vi "Check_Beam_Powers.vi"(3 "Mode":T7, 5 "Traverse line In":T4 {"Carrier_2 Q (l/min)" format="%#.2f"; "Row Duration (mins)" format="%#.1f"; "Row No" min=0; "Trace Gas Concentration (%)" min=0.0 format="%#_4f"; "Carrier_1 Q (l/min)" format="%#.2f"; "Tunnel Speed" format="%#.2f"; "Start X" format="%#.2f"; "Start Y" format="%#.2f"; "Start Z" format="%#.2f"; "End X" format="%#.2f"; "End Y" format="%#.2f"; "End Z" format="%#.2f"; "Averaging time (min)" min=0.0 format="%#.2f"}) -> (0 "Error Message":string, 1 "Status":T3, 2 "Traverse line Out":T4 {"Carrier_2 Q (l/min)" format="%#.2f"; "Row Duration (mins)" format="%#.1f"; "Row No" min=0; "Trace Gas Concentration (%)" min=0.0 format="%#_4f"; "Carrier_1 Q (l/min)" format="%#.2f"; "Tunnel Speed" format="%#.2f"; "Start X" format="%#.2f"; "Start Y" format="%#.2f"; "Start Z" format="%#.2f"; "End X" format="%#.2f"; "End Y" format="%#.2f"; "End Z" format="%#.2f"; "Averaging time (min)" min=0.0 format="%#.2f"})   [LabVIEW 2016]
uses:
  Gen Trav/Traverse_cluster.ctl
  Gen Trav/Spacing.ctl
  Controls/Multi_run_mode.ctl
  Controls/User_Specific_mode.ctl
  Gen Trav/Multi_Run_Status.ctl
  Controls/Beam_Type.ctl
  Gen Trav/Route mapping/Axis.ctl
  Globals/Meas_global.vi
  Globals/Extra_Commands_Global.vi
  Globals/LDA_meas_global_1.vi
panel:
  out "Power Chart":T1(graph)
  out "Light Power":dbl=8.10606551e-08 format="%^#_9e"
  in  "stop":bool
  out "Powers":dbl[](array[numeric]) format="%.1f"
  out "Beam Data":dbl[][](array[numeric]) format="%.1f"
  out "Beam Type":T2 items=["Green Unshifted", "Green Shifted", "Blue Unshifted", "Blue Shifted"]
  # "X                      Y                   Z"
  # "Green Unshifted\nGreen Shifted\nBlue Unshifted\nBlue Shifted"
  # "X           Y            Z"
  # "Start"
  # "End"
  # "X           Y            Z"
  # "Start"
  # "End"
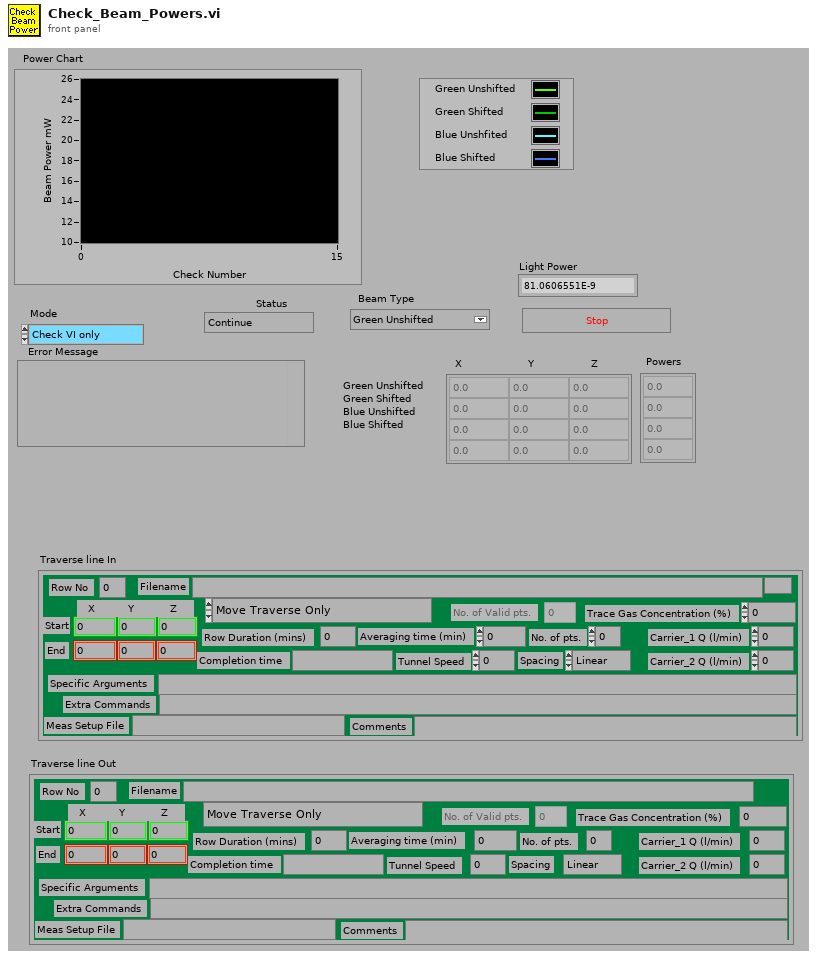
[diagram p1: front panel]
types:
  T1 = cluster{"Numeric":dbl, "Numeric":dbl, "Numeric":dbl, "Numeric":dbl}
  T2 = typedef "Beam_Type.ctl" = u16
  T3 = typedef "Multi_Run_Status.ctl" = enum16{"Continue", "Continue with Error", "Jump to Next Point", "Jump to Next Row", "Jump To Fall Back", "Terminate Run"}
  T4 = typedef "Traverse_cluster.ctl" = cluster{"Start X":sgl, "Start Y":sgl, "Start Z":sgl, "End X":sgl, "End Y":sgl, "End Z":sgl, "No. of pts.":i32, "Spacing":T5, "Filename":path, "Tunnel Speed":dbl, "Averaging time (min)":dbl, "Extra Commands":string, "Carrier_1 Q (l/min)":dbl, "Carrier_2 Q (l/min)":dbl, "Trace Gas Concentration (%)":dbl, "Specific Arguments":string, "Comments":string, "Row No":i32, "Row Type Selector":T6, "Completion time":string, "Row Duration (mins)":dbl, "No. of Valid pts.":i32, "Meas Setup File":string}
  T5 = typedef "Spacing.ctl" = enum16{"Linear", "Log", "Gauss", "Specified", "N/A"}
  T6 = typedef "Multi_run_mode.ctl" = enum16{"Move Traverse Only", "Set Tunnel Speed Only", "Set Source Only", "Set Measurement Conditions", "Single Measurement", "Vertical Profile", "Lateral Profile", "Longitudinal Profile", "Explore Volume", "Multi-Axis Profile", "Auto Calibrate", "Meas Fast FID Bkgnd", "Check Beam Power", "Scanning Valve Measurement", "Run VI Named:", "Set ADAM Ch", "Wait (minutes)", "Send Message", "Synchronize With:", "Fall Back to this Row", "Turn Off Row Repeating", "Blank Row", "Traverse 3D Volume"}
  T7 = typedef "User_Specific_mode.ctl" = enum16{"Check VI only", "Run VI"}
  T8 = enum32{"Bad", "Idle", "Run top level", "Running"}
  T9 = typedef "LDA_Setup.ctl" = cluster{"dimensions":enum16{"1D", "2D"}, "Analogue Freq Multiplier":dbl}
  T10 = enum16{"Load From Excel File", "Save to Excel File"}
  T11 = typedef "Axis.ctl" = enum16{"X Axis", "X Axis -ve", "Y Axis", "Y Axis -ve", "Z Axis", "Z Axis -ve"}
  T12 = typedef "Status_Cluster.ctl" = cluster{"Status":T3, "Error Type":string, "Error Description":string}
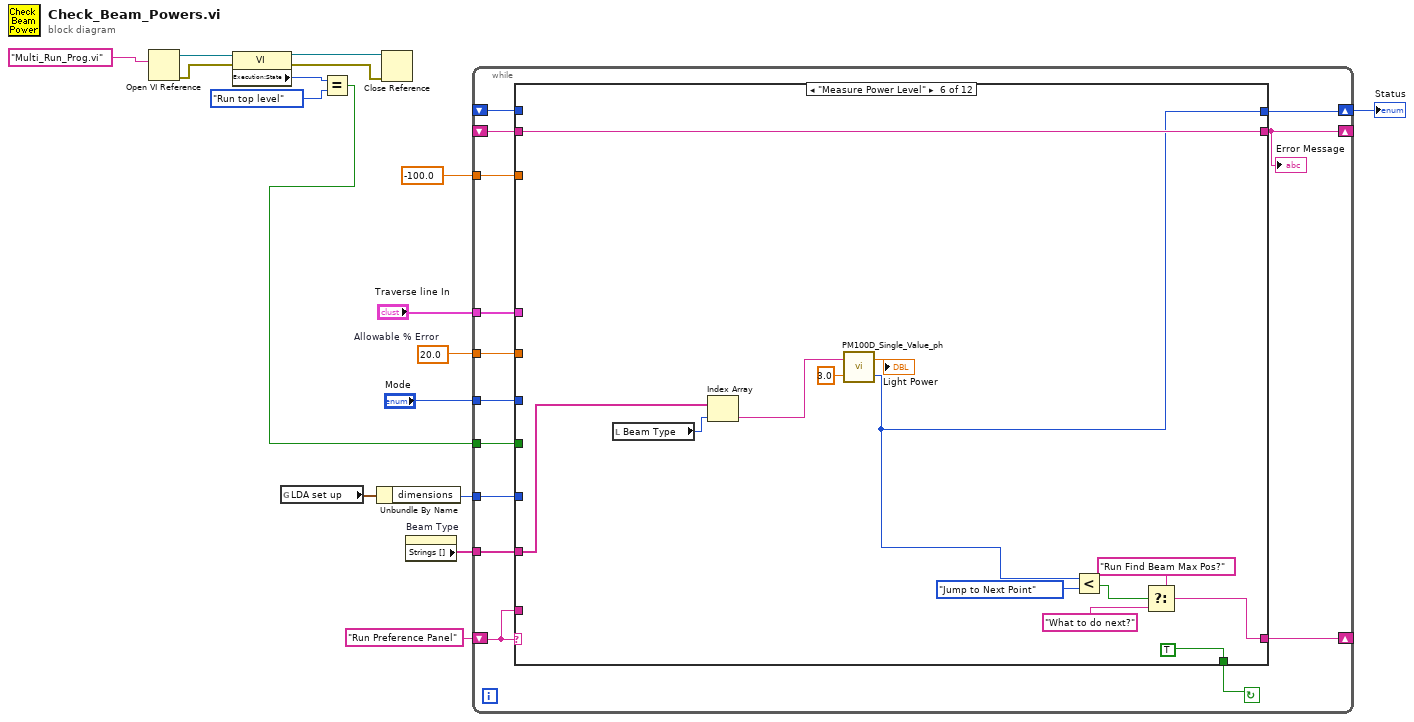
[diagram p0: block diagram]
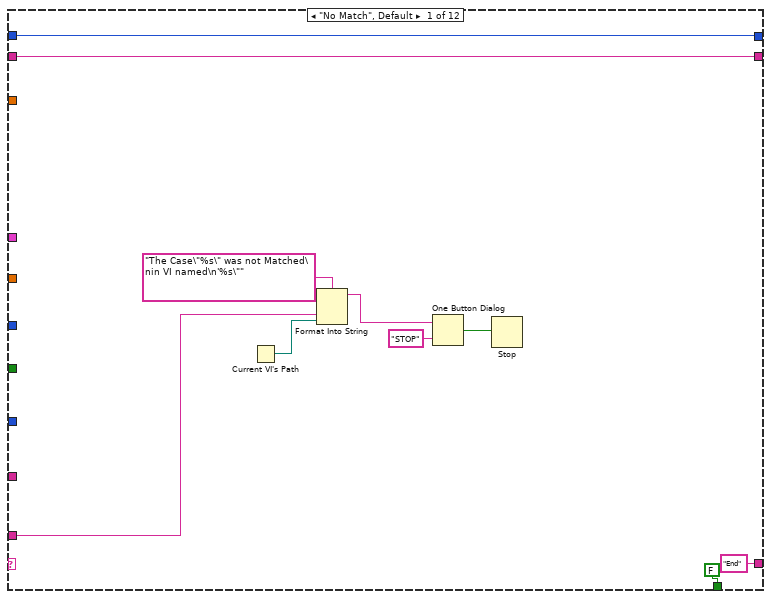
[diagram p2: hidden frame]
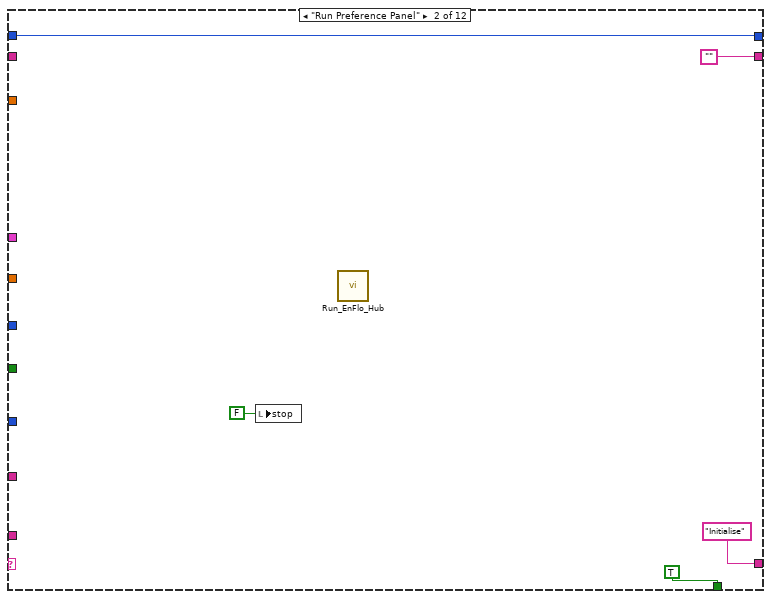
[diagram p3: hidden frame]
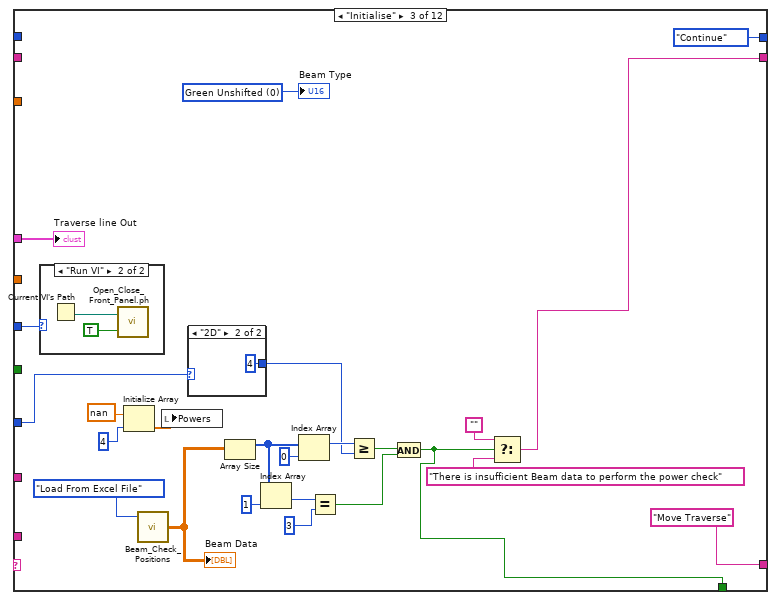
[diagram p4: hidden frame]
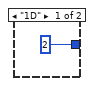
[diagram p5: hidden frame]
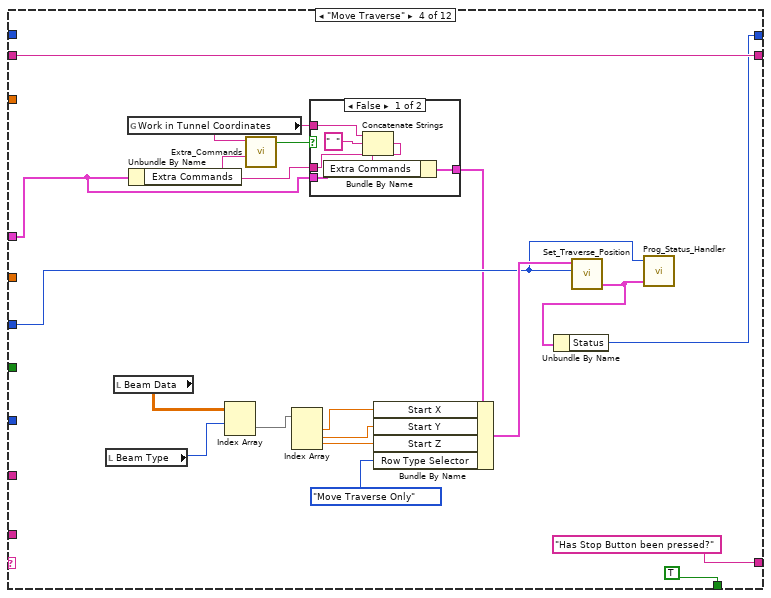
[diagram p7: hidden frame]
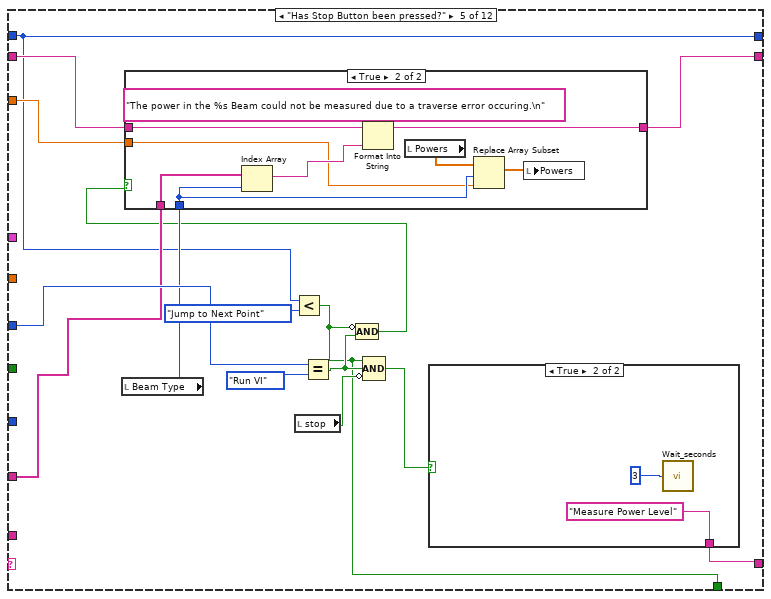
[diagram p9: hidden frame]
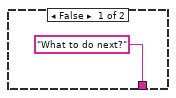
[diagram p11: hidden frame]
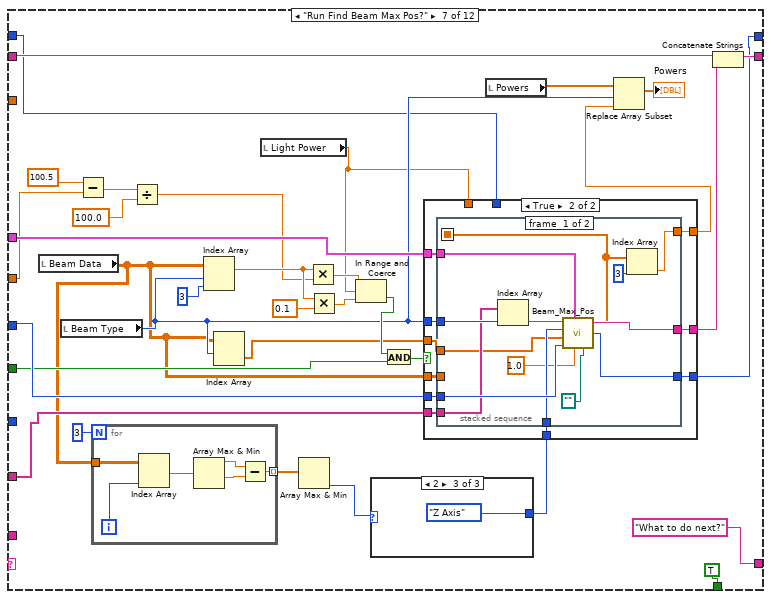
[diagram p12: hidden frame]
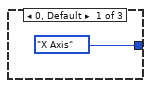
[diagram p13: hidden frame]
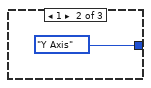
[diagram p14: hidden frame]
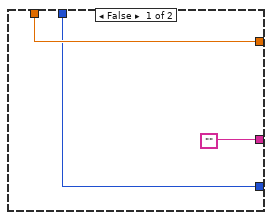
[diagram p15: hidden frame]
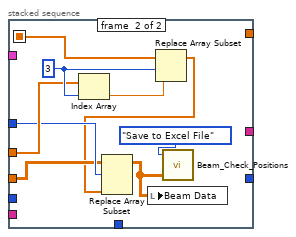
[diagram p16: hidden frame]
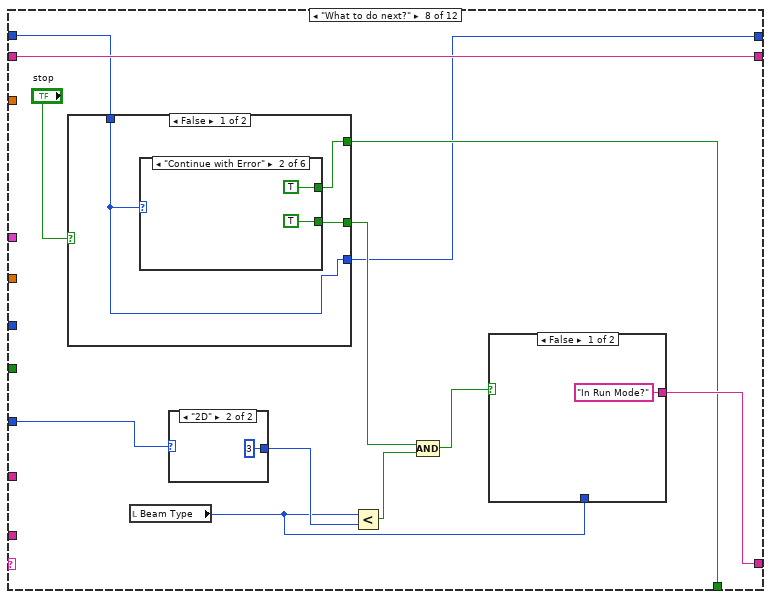
[diagram p17: hidden frame]
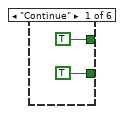
[diagram p18: hidden frame]
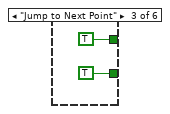
[diagram p19: hidden frame]
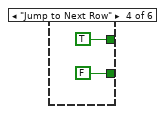
[diagram p20: hidden frame]
diagram:
  w14 = 20.0  # Allowable % Error
  n1 = Open VI Reference(vi path="Multi_Run_Prog.vi") -> (vi reference=w8:refnum<vi>, error out=w9:errorcluster)  [unwired: 1 in, 4 out]
  n2 = property class="VI"(reference=w8, error in=w9) -> (reference out=w10:refnum<vi>, error out=w11:errorcluster, "Execution:State"=w7:T8)
  n3 = global read "Meas_global.vi" "LDA set up"() -> (w2:T9)
  n4 = Equal?(x=w7, y=T8."Run top level" ("Exec.State")) -> (x = y?=w5:bool)
  n5 = Unbundle By Name(w2) -> ("dimensions"=w1:enum16{"1D", "2D"})
  n6 = Close Reference(reference=w10, error in (no error)=w11) -> ()  [unwired: 1 out]
  n7 = property on="Beam Type" class="Ring (strict)"() -> ("Strings []"=w15:string[])  [unwired: 2 in, 2 out]
  n8 = while {
    tunnel: -100.0 ("Element Data") -> [w21]
    tunnel: w14 -> [w23]
    shift-left: _ -> [w25]
    shift-right: [w24] -> _
    tunnel: w1 -> [w26]
    tunnel: w15 -> [w29]
    tunnel: "Traverse line In" -> [w30]
    tunnel: "Mode" -> [w31]
    shift-left: "Run Preference Panel" -> [w22]
    shift-right: [w27] -> _
    tunnel: w5 -> [w20]
    shift-right: [w19] -> w3
    shift-left: _ -> [w18]
    stop <- w28 continue-if-true
    n9 = case shown="\"Measure Power Level\"" w22 {
      tunnel: w30 -> [_ _ w68 w76 _ _ w174 _ _ _ _ _]
      tunnel: w31 -> [_ _ w65 w89 w113 _ w173 _ w261 _ _ _]
      tunnel: w29 -> [_ _ _ _ w111 w131 w148 _ _ w278 _ _]
      tunnel: [FALSE ("Update Datum Powers?") TRUE ("Update Datum Powers?") w47 TRUE w102 TRUE TRUE w223 w257 TRUE w305 FALSE ("Update Datum Powers?")] -> w28
      tunnel: ["End" "Initialise" "Move Traverse" "Has Stop Button been pressed?" w112 w136 "What to do next?" w225 "Are Powers Acceptable?" "Log Beam Power Readings" "Send Error Email" ("f") "End"] -> w27
      tunnel: w26 -> [_ _ w64 _ _ _ _ w231 _ _ _ _]
      tunnel: w25 -> [w33 _ _ w87 w109 w138 w160 w227 w260 w276 w314 w327]
      tunnel: [w33 "" w48 w87 w110 w138 w159 w227 w260 w275 w314 ""] -> w24
      tunnel: w23 -> [_ _ _ _ _ _ w156 _ _ _ _ _]
      tunnel: w22 -> [w36 _ _ _ _ _ _ _ _ _ _ _]
      tunnel: w21 -> [_ _ _ _ w108 _ _ _ _ w273 _ _]
      tunnel: w20 -> [_ _ _ _ _ _ w149 _ _ _ _ _]
      tunnel: [w32 w42 Multi_Run_Status."Continue" ("Status") w84 w101 w133 w143 w221 w259 w272 w315 w323] -> w19
      tunnel: w18 -> [w32 w42 _ _ w101 _ w142 w222 w259 w272 w315 w323]
      frame "No Match", Default {
        n10 = Current VI's Path() -> (path=w37:path)
        n11 = Format Into String(format string="The Case\"%s\" was not Matched\nin VI named\n'%s\"" ("Format String"), w36, w37) -> (resulting string=w40:string)  [unwired: 2 in, 1 out]
        n12 = One Button Dialog(message=w40, button name ("OK")="STOP") -> (true=w38:bool)
        n13 = Stop(stop? (T)=w38) -> ()
      }
      frame "Run Preference Panel" {
        n14 = local write "stop"(FALSE ("stop")) -> ()
        n15 = call "Run_EnFlo_Hub.vi"() -> ()  [unwired: 1 in, 7 out]
      }
      frame "Initialise" {
        w69 = T2 0 items=["Green Unshifted", "Green Shifted", "Blue Unshifted", "Blue Shifted"] ("Beam Type")
        n16 = case shown="\"Run VI\"" w65 {
          frame "Check VI only" {
          }
          frame "Run VI" {
            n17 = Current VI's Path() -> (path=w73:path)
            n18 = call "Open_Close_Front_Panel.ph.vi"("Front Panel Window:Open"=TRUE, "VI path"=w73) -> ()  [unwired: 2 out]
          }
        }
        n19 = Initialize Array(nan ("Numeric"), 4 ("Dimension Size")) -> (w51:dbl[])
        n20 = call "Beam_Check_Positions.vi"("Mode"=T10."Load From Excel File") -> ("Values Out"=w67:dbl[][])  [unwired: 1 in, 1 out]
        "Beam Data" <- w67
        n21 = local write "Powers"(w51) -> ()
        n22 = case shown="\"2D\"" w64 {
          tunnel: [2 4] -> w62
          frame "1D" {
          }
          frame "2D" {
          }
        }
        n23 = Array Size(array=w67) -> (size(s)=w58:i32[])
        n24 = Index Array(array=w58, index=1 ("Index")) -> (element=w57:i32)
        n25 = Index Array(array=w58, index=0 ("Index")) -> (element=w63:i32)
        n26 = Equal?(x=w57, y=3) -> (x = y?=w54:bool)
        n27 = Greater Or Equal?(x=w63, y=w62) -> (x >= y?=w55:bool)
        n28 = And(x=w55, y=w54) -> (x .and. y?=w47:bool)
        n29 = Select(t="", s=w47, f="There is insufficient Beam data to perform the power check") -> (s? t:f=w48:string)
        "Beam Type" <- w69
        "Traverse line Out" <- w68
      }
      frame "Move Traverse" {
        n30 = local read "Beam Type"() -> (w85:T2)
        n31 = local read "Beam Data"() -> (w86:dbl[][])
        n32 = global read "Extra_Commands_Global.vi" "Work in Tunnel Coordinates"() -> (w78:string)
        n33 = Unbundle By Name(w76) -> ("Extra Commands"=w77:string)
        n34 = Index Array(array=w86, index (row)=w85) -> (element=w83:dbl[])  [unwired: 1 in]
        n35 = call "Extra_Commands.vi"("String to Search"=w77, "Command"=w78) -> ("Command Found"=w79:bool)  [unwired: 1 in, 4 out]
        n36 = Index Array(array=w83) -> (element #1=w82:dbl, element #2=w81:dbl, element #3=w80:dbl)  [unwired: 3 in]
        n37 = case shown="False" w79 {
          tunnel: [w99 w100] -> w75
          tunnel: w78 -> [w98 _]
          tunnel: w77 -> [w97 _]
          tunnel: w76 -> [w95 w100]
          frame False {
            n38 = Concatenate Strings(w98, "  " ("string"), w97) -> (w96:string)
            n39 = Bundle By Name(cluster=w95, "Extra Commands"=w96) -> (w99:T4)
          }
          frame True {
          }
        }
        n40 = Bundle By Name(cluster=w75, "Start X"=w82, "Start Y"=w81, "Start Z"=w80, "Row Type Selector"=Multi_run_mode."Move Traverse Only") -> (w92:T4)
        n41 = call "Set_Traverse_Position.vi"("Simulate/Run"=w89, "Traverse line"=w92) -> ("Status Cluster"=w90:T12)  [unwired: 4 in]
        n42 = Unbundle By Name(w90) -> ("Status"=w84:T3)
        n43 = call "Prog_Status_Handler.vi"("Status Cluster"=w90, "Simulate/Run"=w89) -> ()  [unwired: 2 out]
      }
      frame "Has Stop Button been pressed?" {
        n44 = local read "Beam Type"() -> (w107:T2)
        n45 = Less?(x=w101, y=Multi_Run_Status."Jump to Next Point" ("Status")) -> (x < y?=w102:bool)
        n46 = local read "stop"() -> (w106:bool)
        n47 = Equal?(x=w113, y=User_Specific_mode."Run VI" ("Mode")) -> (x = y?=w104:bool)
        n48 = Compound Arithmetic op=AND(invert w102, w104) -> (w103:bool)
        n49 = case shown="True" w103 {
          tunnel: w107 -> [_ w118]
          tunnel: w111 -> [_ w125]
          tunnel: w109 -> [w116 w122]
          tunnel: [w116 w121] -> w110
          tunnel: w108 -> [_ w117]
          frame False {
          }
          frame True {
            n50 = Index Array(array=w125, index=w118) -> (element=w124:string)
            n51 = Format Into String(format string="The power in the %s Beam could not be measured due to a traverse error occuring.\n" ("Format String"), initial string=w122, w124) -> (resulting string=w121:string)  [unwired: 1 in, 1 out]
            n52 = local read "Powers"() -> (w120:dbl[])
            n53 = Replace Array Subset(array=w120, new element=w117, index=w118) -> (w119:dbl[])
            n54 = local write "Powers"(w119) -> ()
          }
        }
        n55 = Compound Arithmetic op=AND(w102, w104, invert w106) -> (w105:bool)
        n56 = case shown="True" w105 {
          tunnel: ["What to do next?" "Measure Power Level"] -> w112
          frame False {
          }
          frame True {
            n57 = call "Wait_seconds.vi"("Seconds to wait"=u32 3) -> ()
          }
        }
      }
      frame "Measure Power Level" {
        n58 = local read "Beam Type"() -> (w132:T2)
        n59 = Index Array(array=w131, index=w132) -> (element=w130:string)
        n60 = call "PM100D_Single_Value_ph.vi"("Averaging Period (s)"=3.0, "Beam Name"=w130) -> ("Status"=w133:T3, "Light Power mW"=→"Light Power":dbl)
        n61 = Less?(x=w133, y=Multi_Run_Status."Jump to Next Point" ("Status")) -> (x < y?=w139:bool)
        n62 = Select(t="Run Find Beam Max Pos?", s=w139, f="What to do next?") -> (s? t:f=w136:string)
      }
      frame "Run Find Beam Max Pos?" {
        n63 = local read "Beam Data"() -> (w145:dbl[][])
        n64 = local read "Beam Type"() -> (w147:T2)
        n65 = Subtract(x=100.5, y=w156) -> (x-y=w155:dbl)
        n66 = for {
          N: 3 -> [_]
          tunnel: w145 -> [w183]
          tunnel: [w179] -> w171 mode=indexing
          i -> [w184]
          n67 = Index Array(array=w183, index (col)=w184) -> (element=w182:dbl[])  [unwired: 1 in]
          n68 = Array Max & Min(array=w182) -> (max value=w181:dbl, min value=w180:dbl)  [unwired: 2 out]
          n69 = Subtract(x=w181, y=w180) -> (x-y=w179:dbl)
        }
        n70 = Divide(x=w155, y=100.0) -> (x/y=w153:dbl)
        n71 = Index Array(array=w145, index (row)=w147, index (col)=3 ("Index")) -> (element=w167:dbl)
        n72 = Index Array(array=w145, index (row)=w147) -> (element=w146:dbl[])  [unwired: 1 in]
        n73 = local read "Light Power"() -> (w144:dbl)
        n74 = Array Max & Min(array=w171) -> (min index (indices)=w170:i32)  [unwired: 3 out]
        n75 = Multiply(x=w167, y=w153) -> (x*y=w165:dbl)
        n76 = Multiply(x=w167, y=0.1) -> (x*y=w164:dbl)
        n77 = In Range and Coerce(upper limit=w165, x=w144, lower limit=w164) -> (In Range?=w151:bool)  [unwired: 1 out]
        n78 = case shown="2" w170 {
          tunnel: [Axis."X Axis" ("Fixed Axis") Axis."Y Axis" ("Fixed Axis") Axis."Z Axis" ("Fixed Axis")] -> w169
          frame 0, Default {
          }
          frame 1 {
          }
          frame 2 {
          }
        }
        n79 = And(x=w151, y=w149) -> (x .and. y?=w150:bool)
        n80 = case shown="True" w150 {
          tunnel: w147 -> [_ w192]
          tunnel: w174 -> [_ w197]
          tunnel: w173 -> [_ w196]
          tunnel: w169 -> [_ w195]
          tunnel: [w187 w194] -> w161
          tunnel: w144 -> [w187 _]
          tunnel: ["" w193] -> w158
          tunnel: w148 -> [_ w191]
          tunnel: w146 -> [_ w190]
          tunnel: w145 -> [_ w189]
          tunnel: [w185 w188] -> w143
          tunnel: w142 -> [w185 _]
          frame False {
          }
          frame True {
            n81 = stacked-sequence {
              seq-local: [w200 _] -> [_ w218]
              tunnel: w197 -> [w211 _]
              tunnel: w196 -> [w210 _]
              tunnel: w195 -> [w209 _]
              tunnel: [w207 _] -> w194
              tunnel: [w206 _] -> w193
              tunnel: w192 -> [w204 w216]
              tunnel: w191 -> [w203 _]
              tunnel: w190 -> [w201 w217]
              tunnel: w189 -> [_ w215]
              tunnel: [w198 _] -> w188
              frame #0 {
                n82 = Index Array(array=w203, index=w204) -> (element=w202:string)
                n83 = call "Beam_Max_Pos.vi"("Picture Log"=path "", "Search Step (mm)"=1.0, "Mode"=w210, "Starting Position"=w201, "Traverse line In"=w211, "Fixed Axis"=w209, "Beam Name"=w202) -> ("Status"=w198:T3, "Beam maxima"=w200:dbl[], "Message"=w206:string)  [unwired: 1 out]
                n84 = Index Array(array=w200, index=3 ("Index")) -> (element=w207:dbl)
              }
              frame #1 {
                w219 = 3 ("index")
                n85 = Index Array(array=w217, index=w219) -> (element=w220:dbl)
                n86 = Replace Array Subset(array=w218, new element=w220, index=w219) -> (w212:dbl[])
                n87 = Replace Array Subset(array=w215, new element=w212, index (row)=w216) -> (w214:dbl[][])  [unwired: 1 in]
                n88 = local write "Beam Data"(w214) -> ()
                n89 = call "Beam_Check_Positions.vi"("Values"=w214, "Mode"=T10."Save to Excel File") -> ()  [unwired: 2 out]
              }
            }
          }
        }
        n90 = local read "Powers"() -> (w163:dbl[])
        n91 = Replace Array Subset(array=w163, new element=w161, index=w147) -> (→"Powers":dbl[])
        n92 = Concatenate Strings(w160, w158) -> (w159:string)
      }
      frame "What to do next?" {
        n93 = case shown="False" "stop" {
          tunnel: [w235 FALSE] -> w224
          tunnel: [w234 FALSE] -> w223
          tunnel: w222 -> [w233 _]
          tunnel: [w233 Multi_Run_Status."Terminate Run" ("Status")] -> w221
          frame False {
            n94 = case shown="\"Continue with Error\"" w233 {
              tunnel: [TRUE TRUE TRUE FALSE FALSE FALSE] -> w235
              tunnel: [TRUE TRUE TRUE TRUE TRUE FALSE] -> w234
              frame "Continue" {
              }
              frame "Continue with Error" {
              }
              frame "Jump to Next Point" {
              }
              frame "Jump to Next Row" {
              }
              frame "Jump To Fall Back" {
              }
              frame "Terminate Run" {
              }
            }
          }
          frame True {
          }
        }
        n95 = local read "Beam Type"() -> (w228:T2)
        n96 = case shown="\"2D\"" w231 {
          tunnel: [1 3] -> w232
          frame "1D" {
          }
          frame "2D" {
          }
        }
        n97 = Less?(x=w228, y=w232) -> (x < y?=w230:bool)
        n98 = Compound Arithmetic op=AND(w224, w230) -> (w229:bool)
        n99 = case shown="False" w229 {
          tunnel: w228 -> [_ w254]
          tunnel: ["In Run Mode?" "Move Traverse"] -> w225
          frame False {
          }
          frame True {
            n100 = Increment(x=w254) -> (x+1=w253:T2)
            n101 = local write "Beam Type"(w253) -> ()
          }
        }
      }
      frame "In Run Mode?" {
        n102 = Equal?(x=w261, y=User_Specific_mode."Run VI" ("Mode")) -> (x = y?=w257:bool)
      }
      frame "Are Powers Acceptable?" {
        n103 = global read "LDA_meas_global_1.vi" "Min Green Unshifted Power mW"() -> (w264:i32)
        n104 = global read "LDA_meas_global_1.vi" "Min Blue Unshifted Power mW"() -> (w266:i32)
        n105 = global read "LDA_meas_global_1.vi" "Min Green Shifted Power mW"() -> (w265:i32)
        n106 = global read "LDA_meas_global_1.vi" "Min Blue Shifted Power mW"() -> (w267:i32)
        n107 = local read "Powers"() -> (w279:dbl[])
        n108 = Build Array(w264, w265, w266, w267) -> (w268:i32[])
        n109 = To Double Precision Float(number=w268) -> (double precision float=w263:dbl[])
        n110 = for {
          tunnel: w279 -> [w286] mode=indexing
          tunnel: w263 -> [w285] mode=indexing
          shift-right: [w295] -> w270
          shift-left: "" -> [w297]
          tunnel: w278 -> [w296] mode=indexing
          tunnel: w273 -> [w290]
          n111 = Subtract(x=w286, y=w285) -> (x-y=w291:dbl)
          n112 = Divide(x=w291, y=w285) -> (x/y=w293:dbl)
          n113 = Not Equal?(x=w290, y=w286) -> (x != y?=w287:bool)
          n114 = Absolute Value(x=w293) -> (abs(x)=w292:dbl)
          n115 = Multiply(x=w292, y=100.0) -> ()  [unwired: 1 out]
          n116 = Less Than 0?(x=w291) -> (x < 0?=w288:bool)
          n117 = Compound Arithmetic op=AND(w287, w288) -> (w289:bool)
          n118 = case shown="True" w289 {
            tunnel: w297 -> [w298 w303]
            tunnel: w296 -> [_ w304]
            tunnel: [w298 w302] -> w295
            tunnel: w286 -> [_ w300]
            tunnel: w285 -> [_ w299]
            frame False {
            }
            frame True {
              n119 = Format Into String(format string="The %s laser beam power is %.1f mW. It lowest acceptable power has been set to %.1f mW. \\n" ("Format String"), initial string=w303, w304, w300, w299) -> (resulting string=w302:string)  [unwired: 1 in, 1 out]
            }
          }
        }
        n120 = Empty String/Path?(string/path=w270) -> (empty?=w271:bool)
        n121 = case shown="False" w271 {
          tunnel: w270 -> [w282 w284]
          tunnel: [w281 w284] -> w269
          frame False {
            n122 = Concatenate Strings(w282, "Please come and check the system As Soon As Possible!\nThe probe may have collided with something or the optical fibres could be getting damaged due to poor launch efficiency! £18,000 TO REPAIR!!\nThe Multi Run will continue." ("Substring")) -> (w281:string)
          }
          frame True {
          }
        }
        n123 = Concatenate Strings(w276, w269) -> (w275:string)
      }
      frame "Log Beam Power Readings" {
        n124 = local read "Powers"() -> (w313:dbl[])
        n125 = local read "Beam Data"() -> (w317:dbl[][])
        n126 = Index Array(array=w313) -> (element #1=w312:dbl, element #2=w311:dbl, element #3=w310:dbl, element #4=w309:dbl)  [unwired: 4 in]
        n127 = Bundle("Numeric"=w312, "Numeric"=w311, "Numeric"=w310, "Numeric"=w309) -> (→"Power Chart":T1)  [unwired: 1 in]
        n128 = for {
          tunnel: w317 -> [w322] mode=indexing
          tunnel: w313 -> [w319] mode=indexing
          tunnel: [w318] -> w316 mode=indexing
          n129 = Array Subset(array=w322, length=3 ("Array Length")) -> (w320:dbl[])  [unwired: 1 in]
          n130 = Build Array (concatenate)(w320, w319) -> (w318:dbl[])
        }
        n131 = Empty String/Path?(string/path=w314) -> (empty?=w306:bool)
        n132 = Not(x=w306) -> (.not. x?=w305:bool)
        n133 = call "Log_beam_power.vi"("Message"=w314, "Beam Data"=w316) -> ()  [unwired: 4 out]
      }
      frame "Send Error Email" {
        w331 = FALSE  # Dialog Box (T)
        n134 = Bundle By Name(cluster=errorcluster {"status"=FALSE, "code"=0, "source"=""} ("error in (no error)"), "source"=w327, "status"=TRUE ("Bundle Element")) -> (w329:errorcluster)
        n135 = call "EnFlo_Error_Handler.vi"("error in (no error)"=w329, "Error Type"="Beam Power", "Dialog Box (T)"=w331) -> ()  [unwired: 3 out]
      }
    }
    "Error Message" <- w24
  }
  "Status" <- w3
